vi "V7310.IO.vi"(6 "timeout ms (5000)":i32=5000, 8 "error in":errorcluster, 10 "Data in":string, 11 "Connection in":refnum<k5>) -> (0 "error out":errorcluster, 1 "Error Level":T1, 2 "Data out":string, 3 "Connection out":refnum<k5>)   [LabVIEW 2016]
uses:
  V7310.ErrorLevels.ctl
panel:
  out "Numeric":i32
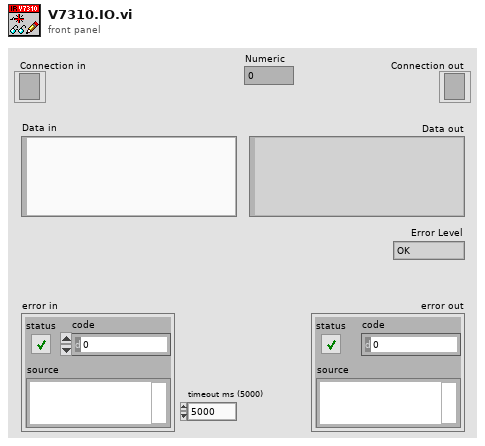
[diagram p1: front panel]
types:
  T1 = typedef "V7310.ErrorLevels.ctl" = enum16{"OK", "Warning", "Error"}
  T2 = enum16{"Standard", "Buffered", "CRLF", "Immediate"}
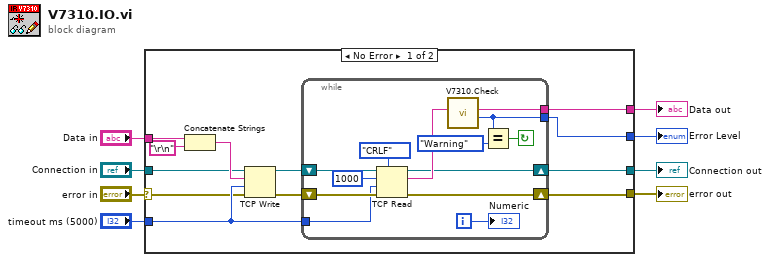
[diagram p0: block diagram]
diagram:
  n1 = case shown="No Error" "error in" {
    selector: "error in" -> [w11 w34]
    tunnel: "Connection in" -> [w12 w35]
    tunnel: [w14 w35] -> w7
    tunnel: "timeout ms (5000)" -> [w17 _]
    tunnel: [w15 w34] -> w3
    tunnel: [w9 _] -> w5
    tunnel: "Data in" -> [w18 _]
    tunnel: [w10 _] -> w1
    frame No Error {
      n2 = Concatenate Strings(w18, "\r\n") -> (w19:string)
      n3 = TCP Write(connection ID=w12, data in=w19, error in (no error)=w11, 9:w17) -> (connection ID out=w16:refnum<k5>, error out=w13:errorcluster)  [unwired: 1 out]
      n4 = while {
        tunnel: [w22] -> w9
        tunnel: [w25] -> w10
        tunnel: w17 -> [w32]
        shift-right: [w28] -> w15
        shift-left: w13 -> [w33]
        shift-right: [w26] -> w14
        shift-left: w16 -> [w31]
        i -> [w21]
        stop <- w23 continue-if-true
        n5 = TCP Read(connection ID=w31, bytes to read=1000, error in (no error)=w33, 7:T2."CRLF" ("mode (standard)"), 9:w32) -> (connection ID out=w26:refnum<k5>, data out=w27:string, error out=w28:errorcluster)
        n6 = call "V7310.Check.vi"("Data in"=w27) -> ("Error Level"=w25:T1, "Data out"=w22:string)  [unwired: 9 in]
        n7 = Equal?(x=w25, y=V7310.ErrorLevels."Warning") -> (x = y?=w23:bool)
        "Numeric" <- w21
      }
    }
    frame Error {
    }
  }
  "Connection out" <- w7
  "error out" <- w3
  "Data out" <- w5
  "Error Level" <- w1
